vi "OAT Remove Duplicate Orders.vi"(1 "array in":dbl[](array[numeric])=[1.0]) -> (0 "array out":dbl[](array[numeric]))   [LabVIEW 2017, in "SoundVib_Gabor.lvlib"]
uses:
  <vilib>/addons/Sound and Vibration/Order Analysis/Gabor Order Tracking/SoundVib_Gabor.lvlib
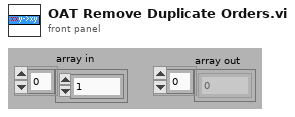
[diagram p1: front panel]
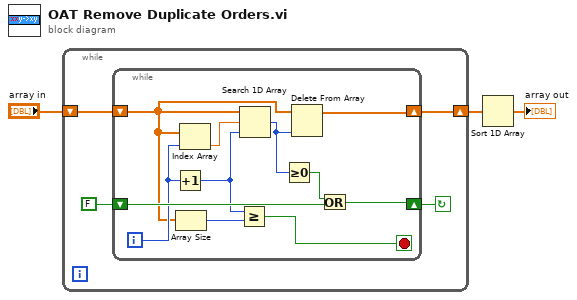
[diagram p0: block diagram]
diagram:
  n1 = while {
    shift-right: [w5] -> w2
    shift-left: "array in" -> [w7]
    stop <- w4 continue-if-true
    n2 = while {
      shift-right: [w18] -> w5
      shift-left: w7 -> [w11]
      shift-right: [w14] -> w4
      shift-left: FALSE -> [w15]
      i -> [w13]
      stop <- w9 stop-if-true
      n3 = Increment(x=w13) -> (x+1=w8:i32)
      n4 = Array Size(array=w11) -> (size(s)=w10:i32)
      n5 = Index Array(array=w11, index=w13) -> (element=w12:dbl)
      n6 = Greater Or Equal?(x=w8, y=w10) -> (x >= y?=w9:bool)
      n7 = Search 1D Array(1D array=w11, element=w12, start index (0)=w8) -> (index of element=w17:i32)
      n8 = Greater Or Equal To 0?(x=w17) -> (x >= 0?=w16:bool)
      n9 = Delete From Array(array=w11, index=w17) -> (array with subset deleted=w18:dbl[])  [unwired: 1 in, 1 out]
      n10 = Or(x=w16, y=w15) -> (x .or. y?=w14:bool)
    }
  }
  n11 = Sort 1D Array(array=w2) -> (sorted array=→"array out":dbl[])
